vi "PathFunctions_RemoveExtension.vi"(0 "Filename":string="aiiiiia.vi", 1 "ExtensionToRemove":string[](array[string])=["vit", "vi"], 5 "ErrorIn":errorcluster) -> (14 "FilenameWithoutExt":string="aiiiiia", 16 "CreatedNewFolder(s)":bool=TRUE, 19 "ErrorOut":errorcluster)   [LabVIEW 2016]
doc: "Entfernt eine bestimmte Fileextension\n\n15.04.14 / sige"
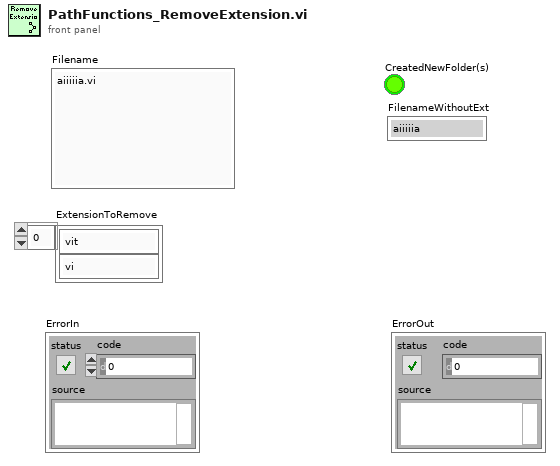
[diagram p1: front panel]
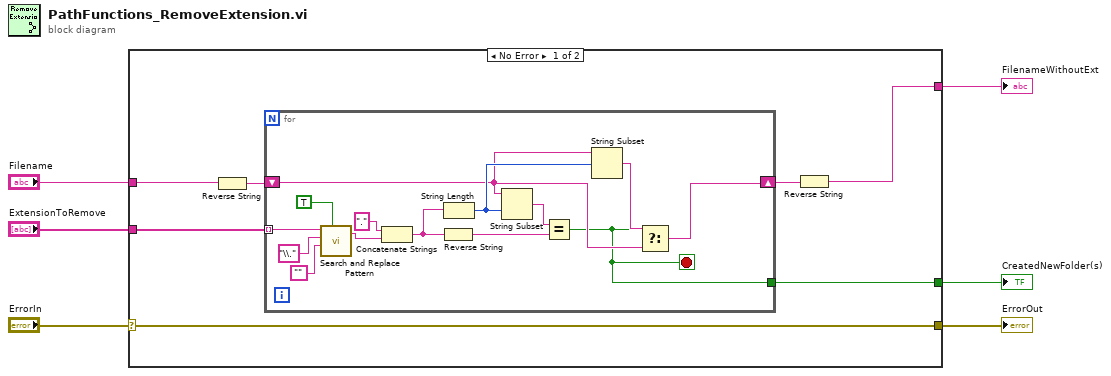
[diagram p0: block diagram]
diagram:
  n1 = case shown="No Error" "ErrorIn" {
    selector: "ErrorIn" -> [w7 w29]
    tunnel: [w7 w29] -> w5
    tunnel: "Filename" -> [w9 w28]
    tunnel: [w10 _] -> w3
    tunnel: [w8 w28] -> w2
    tunnel: "ExtensionToRemove" -> [w13 _]
    frame No Error {
      n2 = Reverse String(1:w9) -> (0:w12:string)
      n3 = for {
        tunnel: w13 -> [w15] mode=indexing
        shift-right: [w18] -> w11
        shift-left: w12 -> [w19]
        tunnel: [w17] -> w10
        stop <- w17 stop-if-true
        n4 = call <vilib>:"Search and Replace Pattern.vi"("string"=w15, "regular expression (\"\")"="\\." ("string"), "replace string (\"\")"="", "replace all? (F)"=TRUE) -> ("result string"=w27:string)  [unwired: 1 in, 1 out]
        n5 = Concatenate Strings("." ("string"), w27) -> (w25:string)
        n6 = Reverse String(1:w25) -> (0:w22:string)
        n7 = String Length(string=w25) -> (length=w21:i32)
        n8 = String Subset(string=w19, length (rest)=w21) -> (substring=w23:string)  [unwired: 1 in]
        n9 = Equal?(x=w23, y=w22) -> (x = y?=w17:bool)
        n10 = String Subset(string=w19, offset (0)=w21) -> (substring=w20:string)  [unwired: 1 in]
        n11 = Select(t=w20, s=w17, f=w19) -> (s? t:f=w18:string)
      }
      n12 = Reverse String(1:w11) -> (0:w8:string)
    }
    frame Error {
    }
  }
  "ErrorOut" <- w5
  "CreatedNewFolder(s)" <- w3
  "FilenameWithoutExt" <- w2
